vi "pidMotor.vi"(6 "output range":cluster{"output high":dbl, "output low":dbl}={"output high"=100.0, "output low"=-100.0} {"output low" format="%.2f"; "output high" format="%.2f"}, 7 "Multiplier":dbl format="%#_13g", 8 "error in (no error)":errorcluster, 9 "PID gains":T1={"proportional gain (Kc)"=1.0, "integral time (Ti, min)"=0.01, "derivative time (Td, min)"=0.0} {"derivative time (Td, min)" format="%.3f"; "integral time (Ti, min)" format="%.3f"; "proportional gain (Kc)" format="%.3f"}, 10 "Joystic  cluster":cluster{"X":dbl, "Y":dbl}, 11 "Encoder":string="My Encoder RefNum") -> (0 "error out":errorcluster, 1 "Rate":dbl, 3 "output":dbl)   [LabVIEW 2013]
uses:
  <vilib>/addons/control/pid/pid.llb/PID Control Input Filter (DBL).vi
  <vilib>/addons/control/pid/pid.llb/PID (DBL).vi
  <vilib>/addons/control/pid/NI_PID_pid.lvlib
  2014DualCanDrive/Reinitializecontrol.ctl
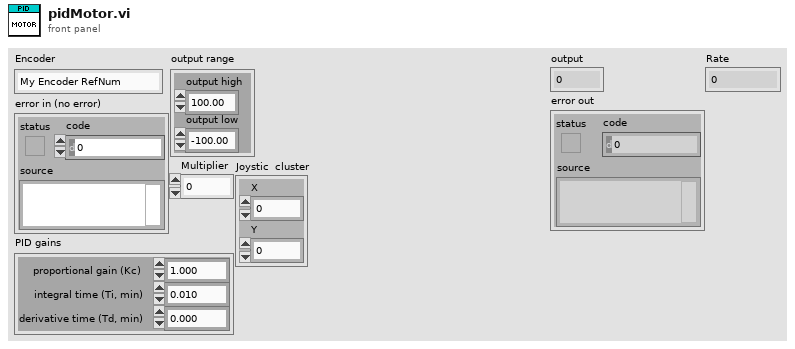
[diagram p1: front panel]
types:
  T1 = cluster{"proportional gain (Kc)":dbl, "integral time (Ti, min)":dbl, "derivative time (Td, min)":dbl}
  T2 = typedef "Reinitializecontrol.ctl" = enum16{"Nonzero", "FollowingZero", "FirstZero"}
  T3 = typedef "WPI_EncoderDevRef.ctl" = cluster{"DevStatus":errorcluster, "EncoderIndex":T4, "CounterIndex":T5, "DistancePerCount":dbl, "Decoding Type":T6}
  T4 = typedef "FPGA_EncoderIdx.ctl" = enum8{"Enc 0", "Enc 1", "Enc 2", "Enc 3", "Invalid"}
  T5 = typedef "FPGA_CounterCtrSystemIndex.ctl" = enum8{"Ctr 0", "Ctr 1", "Ctr 2", "Ctr 3", "Ctr 4", "Ctr 5", "Ctr 6", "Ctr 7", "Invalid"}
  T6 = typedef "WPI_EncoderType.ctl" = enum16{"1x", "2x", "4x"}
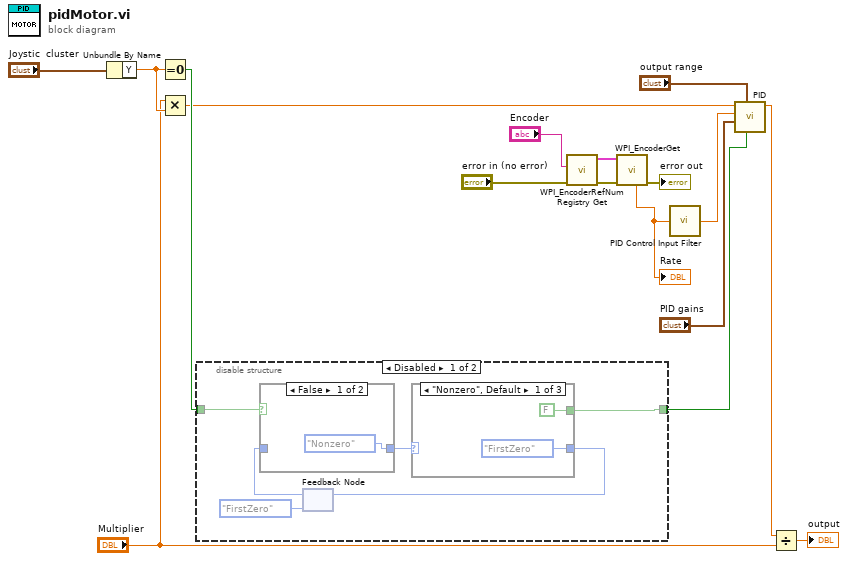
[diagram p0: block diagram]
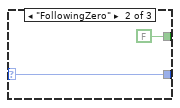
[diagram p3: hidden frame]
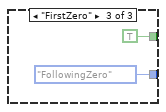
[diagram p4: hidden frame]
diagram:
  n1 = Unbundle By Name("Joystic  cluster") -> ("Y"=w8:dbl)
  n2 = Equal To 0?(x=w8) -> (x = 0?=w11:bool)
  n3 = Multiply(x="Multiplier", y=w8) -> (x*y=w9:dbl)
  n4 = disable-structure shown="Disabled" {
    disable-tunnel: w11 -> [w19 w32]
    disable-tunnel: [w18 w32] -> w10
    frame Disabled {
      n5 = feedback #1(Reinitializecontrol."FirstZero") -> (w21:T2)
      n6 = case shown="False" w19 {
        tunnel: [Reinitializecontrol."Nonzero" w25] -> w22
        tunnel: w21 -> [_ w25]
        frame False {
        }
        frame True {
        }
      }
      n7 = case shown="\"Nonzero\", Default" w22 {
        selector: w22 -> [_ w28 _]
        tunnel: [Reinitializecontrol."FirstZero" w28 Reinitializecontrol."FollowingZero"] -> w20
        tunnel: [FALSE ("reinitialize? (F)") FALSE ("reinitialize? (F)") TRUE ("reinitialize? (F)")] -> w18
        frame "Nonzero", Default {
        }
        frame "FollowingZero" {
        }
        frame "FirstZero" {
        }
      }
      n8 = feedback-in #1(w20) -> ()
    }
    frame Enabled {
    }
  }
  n9 = call <vilib>:"WPI_EncoderRefNum Registry Get.vi"("error in (no error)"="error in (no error)", "refnum name"="Encoder") -> ("error out"=w16:errorcluster, "EncoderDevRef"=w17:T3)  [unwired: 8 in]
  n10 = call <vilib>:"WPI_EncoderGet.vi"("error in (no error)"=w16, "EncoderDevRef"=w17) -> ("error out"=→"error out":errorcluster, "Rate"=w13:dbl)  [unwired: 4 in, 4 out]
  "Rate" <- w13
  n11 = call-poly <vilib>:"PID Control Input Filter.vi"("input"=w13) -> ("output"=w3:dbl)  [unwired: 4 in]
  n12 = call-poly <vilib>:"PID.vi"("reinitialize? (F)"=w10, "output range"="output range", "PID gains"="PID gains", "process variable"=w3, "setpoint"=w9) -> ("output"=w5:dbl)  [unwired: 5 in, 1 out]
  n13 = Divide(x=w5, y="Multiplier") -> (x/y=→"output":dbl)
